vi "Fpga-Top-Level.vi"() -> ()   [LabVIEW 2017]
uses:
  <vilib>/Platform/TimedLoop/XDataNode/timing_clust.ctl
  <vilib>/Platform/TimedLoop/XDataNode/nitl_modes.ctl
  <vilib>/Platform/TimedLoop/XDataNode/wakeup.ctl
  <vilib>/rvi/Emulation/niFpgaSctlEmulationGetInTimedLoop.vi
  <vilib>/rvi/Emulation/niFpgaEmulationReportErrorSimple.vi
  <vilib>/rvi/Emulation/niFpgaGetClockAttributes.vi
  <vilib>/rvi/Emulation/niFpgaCriticalErrorInLSC.vi
  <vilib>/rvi/Emulation/niFpgaEmulationIsFPGAContextNoSignature.vi
  <vilib>/rvi/DataTransferAndStorage/Container/Common/niFpgaContainerGetUniqueNameForEmu.vi
  <vilib>/rvi/Memory/Memory_Emulation/niFpgaMemoryEmulationCacheClearOnFirstRun.vi
  <vilib>/rvi/Memory/Memory_Emulation/nirvimemoryEmulationManagerCache_MakeExclusive.vi
  <vilib>/rvi/Memory/Memory_Emulation/niFpgaMemoryEmulationValidateCache.vi
  <vilib>/rvi/Memory/Memory_Emulation/nirvimemoryEmulationManagerCache_InsertValue.vi
  <vilib>/Utility/error.llb/Clear Errors.vi
  <vilib>/rvi/Memory/Memory_Emulation/nirvimemoryEmulationManagerCache_ReleaseExclusive.vi
  <vilib>/rvi/Memory/Memory_Emulation/nirvimemoryEmulationManagerCache_GetValue.vi
  <vilib>/rvi/Memory/Memory_Emulation/nirvimemoryEmulationManagerCache_SetValue.vi
  <vilib>/rvi/Emulation/niFpgaProcessEmulError.vi
  <vilib>/rvi/interface/RandomDataEmulation/niFpgaRandomDataHandleErrors.vi
  <vilib>/rvi/Memory/Memory_Emulation/niFpgaMemoryFastEmulationDramWriteAndRequestData.vi
  <vilib>/rvi/Memory/Memory_Emulation/niFpgaMemoryEmulationDramWriteAndRequestData.vi
  <vilib>/rvi/Memory/Memory_Emulation/niFpgaMemoryEmulationDramWriteAndRequestDataApplyByteEnables.vi
  <vilib>/rvi/DataTransferAndStorage/Container/Common/niFpgaContainerExecOnDevCompGetState.vi
  <vilib>/Platform/TimedLoop/XDataNode/XDataNode.xnode
  <vilib>/rvi/DataTransferAndStorage/Container/XNode/niFpgaContainer.xnode
  <vilib>/rvi/DataTransferAndStorage/Register/Emulation/niFpgaRegisterEmulation.vi
  <vilib>/rvi/interface/RandomDataEmulation/nirviRandomDataFpgaReadWriteTemplate.vi
  <vilib>/rvi/Memory/Memory_Emulation/niFpgaMemoryEmulationDramRetrieveDataRefIn.vi
  <vilib>/Platform/TimedLoop/XDataNode/XDNodeRunTimeDep.lvlib
panel:
  in  "Size-in":i32
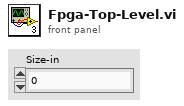
[diagram p1: front panel]
types:
  T1 = typedef "XDNodeRunTimeDep.lvlib/timing_clust.ctl" = cluster{"Expected End [f-1]":u64, "Actual End [f-1]":u64, "Finished Late? [f-1]":bool, "Expected End [i-1]":u64, "Actual End [i-1]":u64, "Finished Late? [i-1]":bool, "Expected Start [i]":u64, "Actual Start [i]":u64, "Expected Start [f]":u64, "Actual Start [f]":u64, "Source Name":string, "Structure Name":string, "Period":i64, "Deadline":i64, "Offset":i64, "Start":i64, "Priority":i32, "Timeout":i32, "Mode":T2, "Wakeup Reason":T3, "Error":errorcluster, "Source Type":string, "Secondary Source Type":string, "Global End Time":u64, "Global Start Time":u64, "Frame Duration":u64, "Iteration Duration":u64, "Assigned CPU":i32, "I/O Scan Engine Mode":u32}
  T2 = typedef "XDNodeRunTimeDep.lvlib/nitl_modes.ctl" = enum32{"No Change", "Process missed periods, maintain original phase", "Discard missed periods, maintain original phase", "Process missed periods, ignore original phase", "Discard missed periods, ignore original phase"}
  T3 = typedef "XDNodeRunTimeDep.lvlib/wakeup.ctl" = enum32{"Normal", "Aborted", "Asynchronous wakeup", "Timing source error", "Timed loop error", "Timeout"}
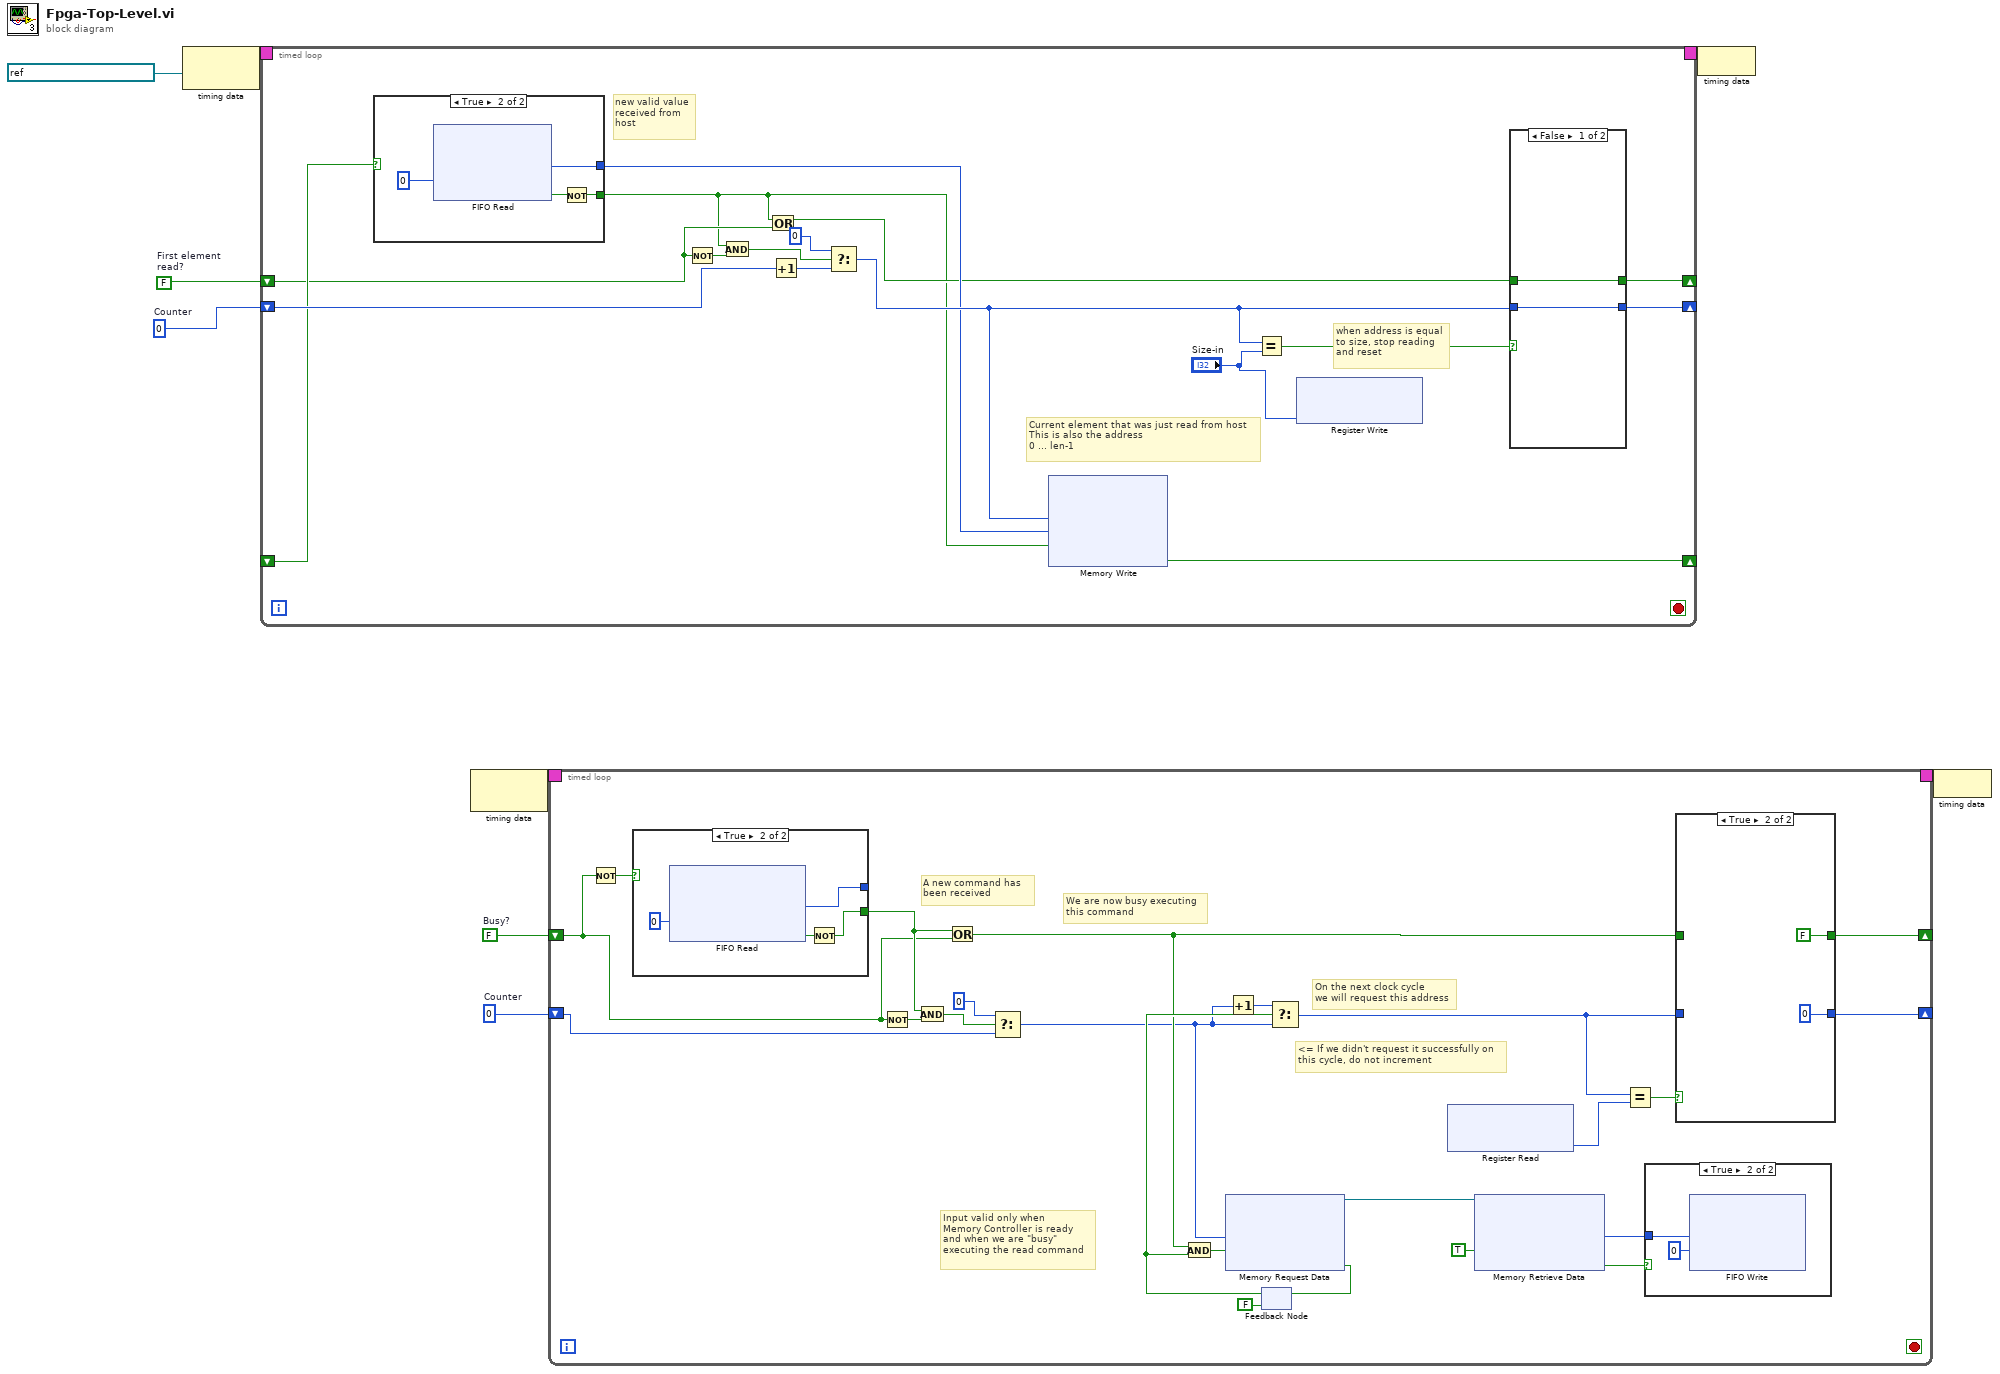
[diagram p0: block diagram]
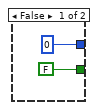
[diagram p4: hidden frame]
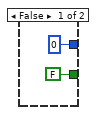
[diagram p5: hidden frame]
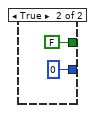
[diagram p6: hidden frame]
diagram:
  w1 = i16 0  # Counter
  w2 = FALSE  # Busy?
  w6 = FALSE  # First element read?
  w5 = i16 0  # Counter
  n1 = node-c288(refnum<k21> "40 MHz Onboard Clock" ("Source Name")) -> (w9:T1)
  n2 = timed-loop {
    timing: w9 -> [_]
    timing-out: [_] -> w8
    shift-right: [w25] -> _
    shift-left: w6 -> [w13]
    shift-right: [w24] -> _
    shift-left: w5 -> [w21]
    shift-right: [w10] -> _
    shift-left: _ -> [w17]
    stop <- _ stop-if-true
    # "when address is equal\nto size, stop reading\nand reset"
    # "Current element that was just read from host\nThis is also the address\n0 ... len-1"
    # "new valid value\nreceived from\nhost"
    n3 = case shown="True" w17 {
      tunnel: [FALSE w29] -> w11
      tunnel: [u8 0 ("Element") w28] -> w15
      frame False {
      }
      frame True {
        n4 = xnode "FIFO Read"("Timeout"=0) -> ("Element"=w28:u8, "Timed Out?"=w30:bool)  [unwired: 1 in, 1 out]
        n5 = Not(x=w30) -> (.not. x?=w29:bool)
      }
    }
    n6 = Not(x=w13) -> (.not. x?=w23:bool)
    n7 = And(x=w11, y=w23) -> (x .and. y?=w19:bool)
    n8 = Or(x=w11, y=w13) -> (x .or. y?=w14:bool)
    n9 = Increment(x=w21) -> (x+1=w22:i16)
    n10 = Select(t=i16 0, s=w19, f=w22) -> (s? t:f=w16:i16)
    n11 = xnode "Memory Write"("Address"=w16, "Data"=w15, "Input Valid"=w11) -> ("Ready for Input"=w10:bool)  [unwired: 1 in, 1 out]
    n12 = Equal?(x=w16, y="Size-in") -> (x = y?=w18:bool)
    n13 = xnode "Register Write"("Data"="Size-in") -> ()  [unwired: 1 in, 1 out]
    n14 = case shown="False" w18 {
      tunnel: w14 -> [w33 _]
      tunnel: w16 -> [w32 _]
      tunnel: [w33 FALSE ("Reading?")] -> w25
      tunnel: [w32 i16 0 ("t")] -> w24
      frame False {
      }
      frame True {
      }
    }
  }
  n15 = node-c288() -> (w4:T1)  [unwired: 1 in]
  n16 = timed-loop {
    timing: w4 -> [_]
    timing-out: [_] -> w3
    shift-right: [w59] -> _
    shift-left: w2 -> [w53]
    shift-right: [w52] -> _
    shift-left: w1 -> [w55]
    stop <- _ stop-if-true
    # "Input valid only when\nMemory Controller is ready\nand when we are \"busy\"\nexecuting the read command"
    # "<= If we didn't request it successfully on\nthis cycle, do not increment"
    # "On the next clock cycle\nwe will request this address"
    # "We are now busy executing\nthis command"
    # "A new command has\nbeen received"
    n17 = Not(x=w53) -> (.not. x?=w60:bool)
    n18 = case shown="True" w60 {
      tunnel: [FALSE w70] -> w54
      tunnel: [u32 0 ("Element") w69] -> _
      frame False {
      }
      frame True {
        n19 = xnode "FIFO Read"("Timeout"=0) -> ("Element"=w69:u32, "Timed Out?"=w71:bool)  [unwired: 1 in, 1 out]
        n20 = Not(x=w71) -> (.not. x?=w70:bool)
      }
    }
    n21 = Not(x=w53) -> (.not. x?=w58:bool)
    n22 = And(x=w54, y=w58) -> (x .and. y?=w56:bool)
    n23 = Or(x=w54, y=w53) -> (x .or. y?=w44:bool)
    n24 = Select(t=i16 0, s=w56, f=w55) -> (s? t:f=w38:i16)
    n25 = Increment(x=w38) -> (x+1=w43:i16)
    n26 = feedback #1(FALSE ("Ready for Input")) -> (w48:bool)
    n27 = And(x=w44, y=w48) -> (x .and. y?=w39:bool)
    n28 = xnode "Memory Request Data"("Address"=w38, "Input Valid"=w39) -> ("Ready for Input"=w50:bool, "Memory Out"=w45:refnum<k21>)  [unwired: 1 in]
    n29 = feedback-in #1(w50) -> ()
    n30 = Select(t=w43, s=w48, f=w38) -> (s? t:f=w42:i16)
    n31 = xnode "Register Read"() -> ("Data"=w41:u32)  [unwired: 1 in, 1 out]
    n32 = xnode "Memory Retrieve Data"("Ready for Output"=TRUE, "Memory In"=w45) -> ("Data"=w47:u8, "Output Valid"=w40:bool)  [unwired: 1 out]
    n33 = Equal?(x=w42, y=w41) -> (x = y?=w51:bool)
    n34 = case shown="True" w40 {
      tunnel: w47 -> [_ w62]
      frame False {
      }
      frame True {
        n35 = xnode "FIFO Write"("Element"=w62, "Timeout"=0) -> ()  [unwired: 1 in, 2 out]
      }
    }
    n36 = case shown="True" w51 {
      tunnel: [w64 FALSE] -> w59
      tunnel: w44 -> [w64 _]
      tunnel: [w63 i16 0 ("t")] -> w52
      tunnel: w42 -> [w63 _]
      frame False {
      }
      frame True {
      }
    }
  }
  n37 = node-c288(w8) -> ()
  n38 = node-c288(w3) -> ()
